vi "Register Set Create Sensor Key Focus.vi"(8 "error in (no error)":errorcluster, 9 "Data Message":refnum<class "Data Message.lvclass">, 10 "View Enqueuer":refnum<class "Message Enqueuer.lvclass">, 11 "Create Sensor Model in":refnum<class "Create Sensor Model.lvclass">) -> (0 "error out":errorcluster, 3 "Create Sensor Model out":refnum<class "Create Sensor Model.lvclass">)   [LabVIEW 2013, in "Create Sensor Model.lvlib" / "Create Sensor Model.lvclass"]
uses:
  Create Sensor Model.lvclass
  <vilib>/ActorFramework/Message Enqueuer/Message Enqueuer.lvclass
  <vilib>/ActorFrameworkMVC/View Observer/Data Message/Data Message.lvclass
  Create Sensor Model.lvclass/Create Sensor Model.ctl
  <vilib>/ActorFrameworkMVC/View Observer/View Registry/View Registry.lvclass
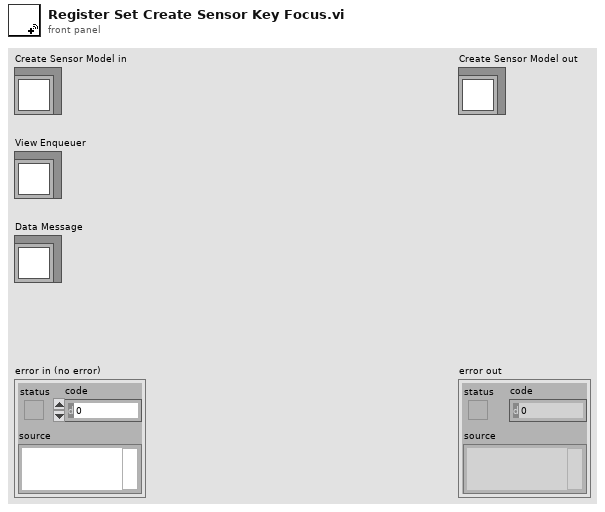
[diagram p1: front panel]
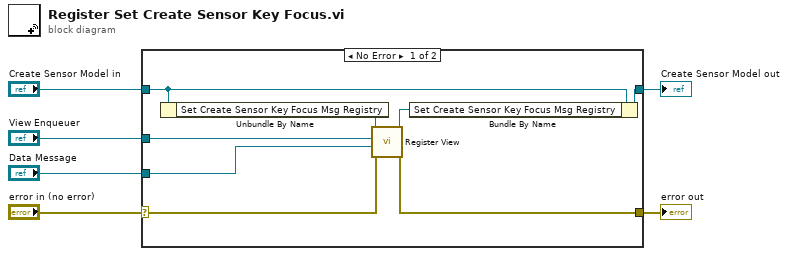
[diagram p0: block diagram]
diagram:
  n1 = case shown="No Error" "error in (no error)" {
    selector: "error in (no error)" -> [w12 w16]
    tunnel: "View Enqueuer" -> [w14 _]
    tunnel: "Create Sensor Model in" -> [w8 w15]
    tunnel: "Data Message" -> [w13 _]
    tunnel: [w7 w15] -> w2
    tunnel: [w11 w16] -> w1
    frame No Error {
      n2 = Unbundle By Name(w8) -> ("Set Create Sensor Key Focus Msg Registry"=w10:refnum<class "View Registry.lvclass">)
      n3 = call <vilib>:"Register View.vi"("error in (no error)"=w12, "Data Message"=w13, "View Enqueuer"=w14, "View Registry in"=w10) -> ("error out"=w11:errorcluster, "View Registry out"=w9:refnum<class "View Registry.lvclass">)  [unwired: 6 in]
      n4 = Bundle By Name(cluster=w8, "Set Create Sensor Key Focus Msg Registry"=w9) -> (w7:refnum<class "Create Sensor Model.lvclass">)
    }
    frame Error {
    }
  }
  "error out" <- w1
  "Create Sensor Model out" <- w2
